vi "GVaktuelleTDMS.vi"() -> ()   [LabVIEW 2017]
panel:
  out "aktuelleTDMS-DateiECD2":refnum<k34>
  out "aktuelleTDMS-DateiECD1":refnum<k34>
  out "aktuelleTDMS-DateiHK":refnum<k34>
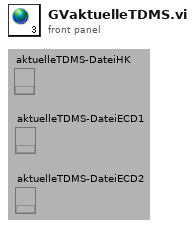
[diagram p1: front panel]
diagram:
